vi "Undo Servo.vi"(7 "Description":string, 8 "Command Info In":T1, 9 "Ratchet":bool, 10 "Activation?":bool, 11 "Motor power":dbl) -> (0 "Command Info Out":T1)   [LabVIEW 2019]
doc: "This template is useful for immediate subsystem actions that do not need deadband filtering\n\nBe sure to right-click and select New from Template and save with a new command name."
uses:
  <vilib>/Rock Robotics/WPI/Framework/Command Status Info.ctl
  <vilib>/Rock Robotics/WPI/Framework/Completion Status.ctl
  <vilib>/Rock Robotics/WPI/Framework/Completion Notifier.ctl
  Implementation/Hang Setpoints.ctl
  Implementation/Hang Operations.ctl
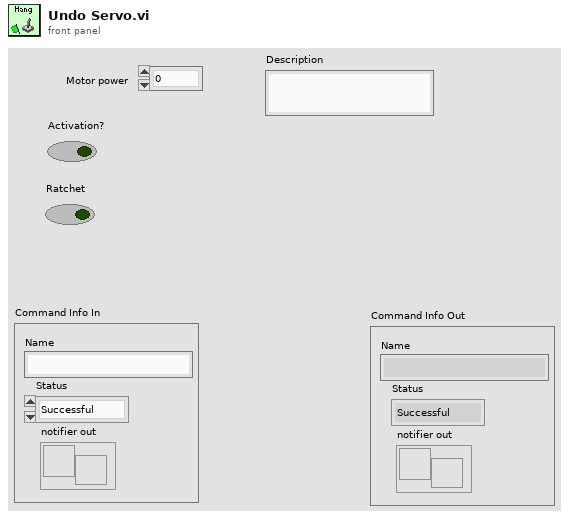
[diagram p1: front panel]
types:
  T1 = typedef "Command Status Info.ctl" = cluster{"Name":string, "Status":T2, "notifier out":T3}
  T2 = typedef "Completion Status.ctl" = enum16{"Successful", "Aborted", "Incomplete"}
  T3 = typedef "Completion Notifier.ctl" = refnum<notifier>
  T4 = typedef "Hang Setpoints.ctl" = cluster{"Operation":T5, "Motor power":dbl, "Activation?":bool, "Ratchet":bool, "Duration":dbl}
  T5 = typedef "Hang Operations.ctl" = enum16{"Reserve", "Read Current", "Immediate", "Undo Ratchet", "Redo Ratchet", "Retract Hang", "Raise Hang"}
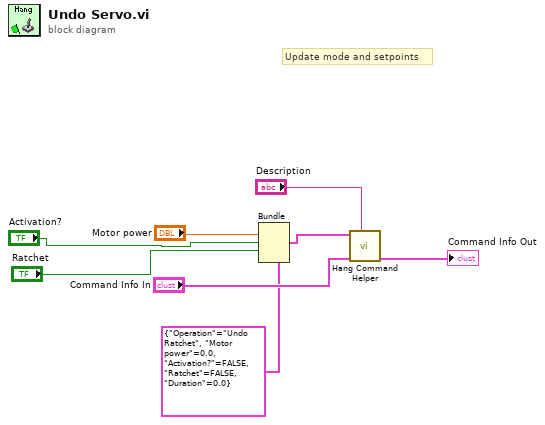
[diagram p0: block diagram]
diagram:
  # "Update mode and setpoints"
  n1 = Bundle(cluster=T4 {"Operation"=enum."Undo Ratchet", "Motor power"=0.0, "Activation?"=FALSE, "Ratchet"=FALSE, "Duration"=0.0} ("SubSystem Data"), "Motor power"="Motor power", "Activation?"="Activation?", "Ratchet"="Ratchet") -> (w1:T4)  [unwired: 2 in]
  n2 = call "Hang Command Helper.vi"("Description"="Description", "Command Info In"="Command Info In", "SubSystem Data"=w1) -> ("Command Info Out"=→"Command Info Out":T1)  [unwired: 6 in, 2 out]
